vi "Tosca-Restore AI Layout.vi"(0 "VI in":refnum<vi>, 5 "GraphSplitter":refnum<vi>, 7 "more in":bool, 11 "error in (no error)":errorcluster) -> (8 "more out":bool, 15 "error out":errorcluster)   [LabVIEW 2020]
uses:
  <vilib>/Utility/miscctls.llb/LVRectTypeDef.ctl
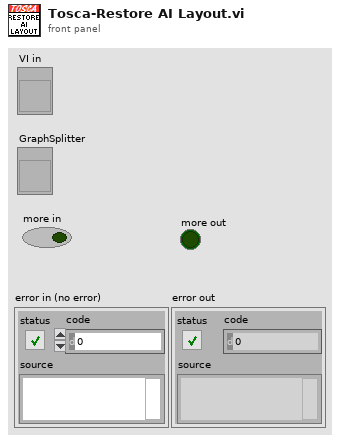
[diagram p1: front panel]
types:
  T1 = typedef "LVRectTypeDef.ctl" = cluster{"Left":i16, "Top":i16, "Right":i16, "Bottom":i16}
  T2 = cluster{"bounds":T1, "splitter":i32, "more":bool}
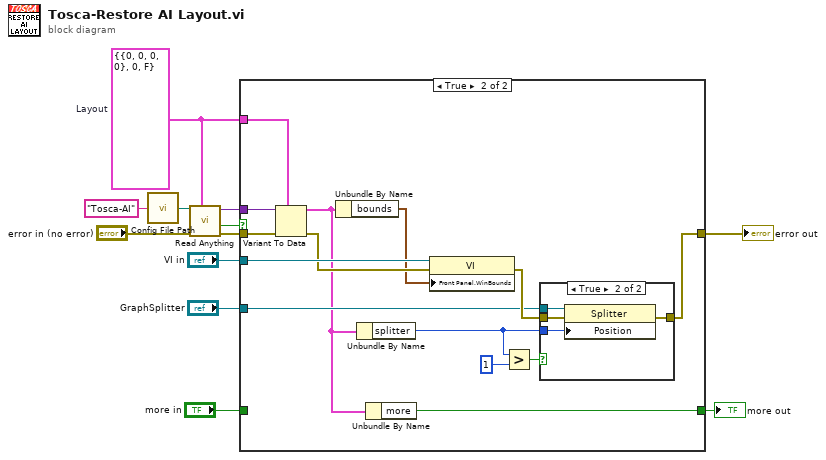
[diagram p0: block diagram]
diagram:
  w7 = T2 {"bounds"={"Left"=0, "Top"=0, "Right"=0, "Bottom"=0}, "splitter"=0, "more"=FALSE}  # Layout
  n1 = call "Config File Path.vi"("AppName"="Tosca-AI") -> ("Default config file name"=w11:path)
  n2 = call "Read Anything.vi"("Type of Anything"=w7, "Error In"="error in (no error)", "Path (dialog)"=w11) -> ("Error Out"=w9:errorcluster, "Found?"=w6:bool, "Anything"=w8:variant)  [unwired: 6 in]
  n3 = case shown="True" w6 {
    tunnel: w9 -> [w14 w28]
    tunnel: w8 -> [_ w27]
    tunnel: w7 -> [_ w26]
    tunnel: "VI in" -> [_ w25]
    tunnel: [w14 w15] -> w4
    tunnel: "GraphSplitter" -> [_ w20]
    tunnel: "more in" -> [w13 _]
    tunnel: [w13 w16] -> w1
    frame False {
    }
    frame True {
      n4 = Variant To Data(error in=w28, type=w26, Variant=w27) -> (data=w17:T2, error out=w24:errorcluster)
      n5 = Unbundle By Name(w17) -> ("bounds"=w23:T1)
      n6 = Unbundle By Name(w17) -> ("splitter"=w18:i32)
      n7 = Unbundle By Name(w17) -> ("more"=w16:bool)
      n8 = property class="VI"(reference=w25, error in=w24, "Front Panel.WinBounds"=w23) -> (error out=w21:errorcluster)  [unwired: 1 out]
      n9 = Greater?(x=w18, y=1) -> (0:w19:bool)
      n10 = case shown="True" w19 {
        tunnel: w21 -> [w29 w33]
        tunnel: w20 -> [_ w32]
        tunnel: w18 -> [_ w31]
        tunnel: [w29 w30] -> w15
        frame False {
        }
        frame True {
          n11 = property class="Splitter"(reference=w32, error in=w33, "Position"=w31) -> (error out=w30:errorcluster)  [unwired: 1 out]
        }
      }
    }
  }
  "error out" <- w4
  "more out" <- w1
